vi "can_receive.vi"() -> ()   [LabVIEW 2009]
panel:
  in  "BTR 1":u32=28 caption="BTR1" format="%x"
  in  "BTR 0":u32=3 caption="BTR0" format="%x"
  in  "K":u16(ring)=1000 items=["10"=10, "20"=20, "50"=50, "100"=100, "125"=125, "250"=250, "500"=500, "800"=800, "1000"=1000]
  in  "Baudrate":enum32{"Standard", "Custom"}(radio)
  out "Received MSG":string[][](table)
  in  "Data Format":enum32{"Hexadecimal", "Decimal"}(radio)
  out "Error out":errorcluster {"code" format="%.0x"}
  in  "NumbertoRead":u32=100
  in  "CANPort":string(combo)="CAN1"
  in  "ReadTimeOut":u32=3000 caption="ms"
  in  "Synchronization":i32(ring)=1 items=["Synchronization"=1, "Asynchronization"=0]
  in  "stop":bool
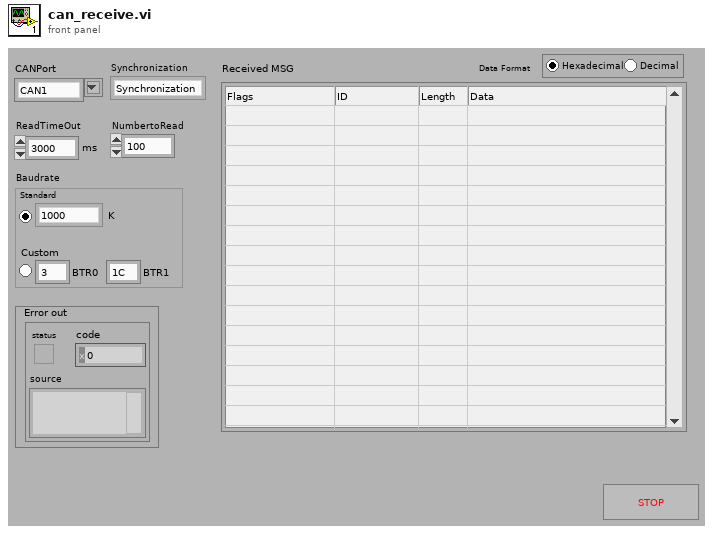
[diagram p1: front panel]
types:
  T1 = cluster{"Internal":u32, "InternalHigh":u32, "Offset":u32, "OffsetHigh":u32, "hEvent":u32}
  T2 = cluster{"Flags":u32, "ID(HEX)":u32, "Length":i16, "Data":u8[]}[]
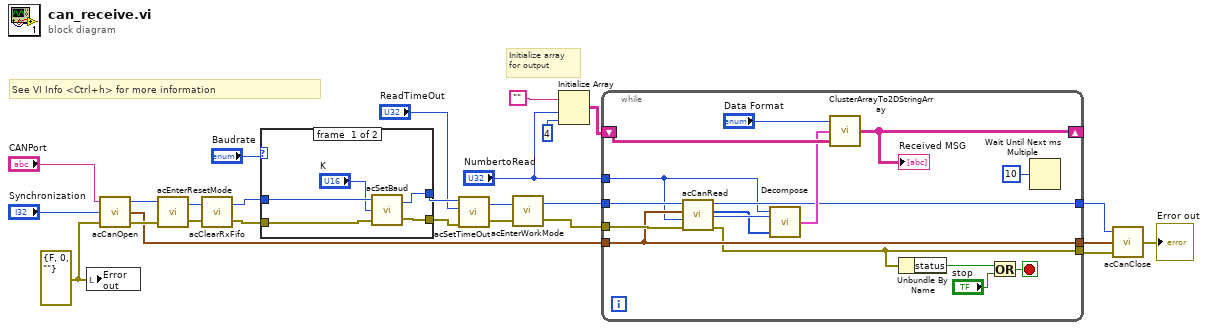
[diagram p0: block diagram]
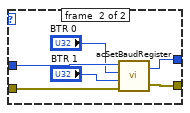
[diagram p2: hidden frame]
diagram:
  w19 = errorcluster {"status"=FALSE, "code"=0, "source"=""} ("Error in")
  # "See VI Info <Ctrl+h> for more information"
  # "Initialize array \nfor output"
  n1 = local write "Error out"(w19) -> ()
  n2 = call "acCanOpen.vi"("Error in"=w19, "Synchronization"="Synchronization", "CANPort"="CANPort") -> ("Error out"=w21:errorcluster, "Overlapped"=w5:T1, "Handle"=w22:u32)
  n3 = call "acEnterResetMode.vi"("Error in"=w21, "Handle  in"=w22) -> ("Error out"=w14:errorcluster, "Handle out"=w13:u32)
  n4 = call "acClearRxFifo.vi"("Error in"=w14, "Handle  in"=w13) -> ("Error out"=w11:errorcluster, "Handle out"=w12:u32)
  n5 = case shown="\"Custom\"" "Baudrate" {
    tunnel: [w30 w37] -> w16
    tunnel: [w31 w36] -> w17
    tunnel: w12 -> [w29 w34]
    tunnel: w11 -> [w28 w35]
    frame #0 {
      n6 = call "acSetBaud.vi"("Error in"=w28, "Baudrate"="K", "Handle  in"=w29) -> ("Error out"=w30:errorcluster, "Handle out"=w31:u32)
    }
    frame #1 {
      n7 = call "acSetBaudRegister.vi"("Error in"=w35, "BTR 1"="BTR 1", "BTR 0"="BTR 0", "Handle  in"=w34) -> ("Error out"=w37:errorcluster, "Handle out"=w36:u32)
    }
  }
  n8 = call "acSetTimeOut.vi"("Error in"=w16, "Read TimeOut"="ReadTimeOut", "Handle  in"=w17) -> ("Error out"=w8:errorcluster, "Handle out"=w9:u32)  [unwired: 1 in]
  n9 = call "acEnterWorkMode.vi"("Error in"=w8, "Handle  in"=w9) -> ("Error out"=w6:errorcluster, "Handle out"=w7:u32)
  n10 = Initialize Array("", "NumbertoRead", 4 ("Dimension Size")) -> (w2:string[][])
  n11 = while {
    tunnel: w7 -> [w51]
    tunnel: w6 -> [w52]
    tunnel: [w48] -> w23
    tunnel: [w40] -> w25
    tunnel: w5 -> [w49]
    tunnel: [w49] -> w24
    shift-right: [w50] -> _
    shift-left: w2 -> [w44]
    tunnel: "NumbertoRead" -> [w38]
    stop <- w42 stop-if-true
    n12 = call "acCanRead.vi"("Error in"=w52, "ReadCount"=w38, "Overlapped"=w49, "Handle  in"=w51) -> ("Error out"=w48:errorcluster, "NumberOfRead"=w46:u32, "MSG"=w45:u8[], "Handle out"=w40:u32)
    n13 = call "Decompose.vi"("Array"=w45, "Real"=w46, "Expect"=w38) -> ("MSG"=w43:T2)
    n14 = call "ClusterArrayTo2DStringArray.vi"("Input Array"=w44, "MSG"=w43, "Data Format"="Data Format") -> ("Output Array"=w50:string[][])
    "Received MSG" <- w50
    n15 = Unbundle By Name(w48) -> ("status"=w41:bool)
    n16 = Or(x=w41, y="stop") -> (x .or. y?=w42:bool)
    n17 = Wait Until Next ms Multiple(millisecond multiple=u32 10) -> ()  [unwired: 1 out]
  }
  n18 = call "acCanClose.vi"("Error in"=w23, "Overlapped"=w24, "Handle  in"=w25) -> ("Error out"=→"Error out":errorcluster)
